vi "ltm4676a_set_runtime_config.vi"(0 "LTM4676A Runtime Config":T1={"SDC config path"=path "C:/Users/Administrator/Documents/qkocian-sandbox/demos/argus-buck-demo/instrumentstudio/sdc/pmbus_ltm4676a.sdconfig", "Output setpoint (V)"=3.3, "Voltage margin (%)"=5.0, "Voltage warn limit (%)"=7.5, "Voltage fault limit (%)"=10.0, "Switching frequency (kHz)"=650} {"Switching frequency (kHz)" items=["250"=62440, "350"=64188, "425"=64338, "500"=64488, "575"=575, "650"=650, "750"=750, "1000"=1000]; "Voltage fault limit (%)" min=0.0 max=100.0 step=1.0 format="%.1g"; "Voltage warn limit (%)" min=0.0 max=100.0 step=1.0 format="%.1g"; "Voltage margin (%)" min=0.0 max=100.0 step=1.0 format="%.1g"; "Output setpoint (V)" min=0.5 max=5.5 step=0.1}, 1 "error in (no error)":errorcluster) -> (2 "Device Control session out":refnum<class "Semiconductor Device Control.lvclass">, 3 "success?":bool, 4 "error out":errorcluster)   [LabVIEW 2021]
uses:
  <instrlib>/Semi Device Control/Semiconductor Device Control.lvclass
  controls/ltm4676a_config.ctl
  controls/ltm4676a_reg_u8.ctl
  controls/ltm4676a_reg_uids.ctl
  controls/ltm4676a_reg_u16.ctl
  <instrlib>/Semi Device Control/API/Instantiate - using IS config path.vi
  <instrlib>/Semi Device Control/API/Start.vi
  <instrlib>/Semi Device Control/API/Stop.vi
  <instrlib>/Semi Device Control/API/Destroy.vi
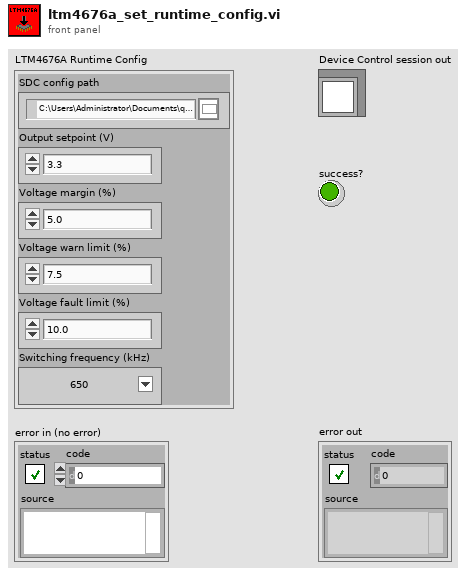
[diagram p1: front panel]
types:
  T1 = typedef "ltm4676a_config.ctl" = cluster{"SDC config path":path, "Output setpoint (V)":dbl, "Voltage margin (%)":dbl, "Voltage warn limit (%)":dbl, "Voltage fault limit (%)":dbl, "Switching frequency (kHz)":u16}
  T2 = typedef "ltm4676a_reg_uids.ctl" = string
  T3 = typedef "ltm4676a_reg_u8.ctl" = cluster{"uid":T2, "val":u8}
  T4 = typedef "ltm4676a_reg_u16.ctl" = cluster{"uid":T2, "val":u16}
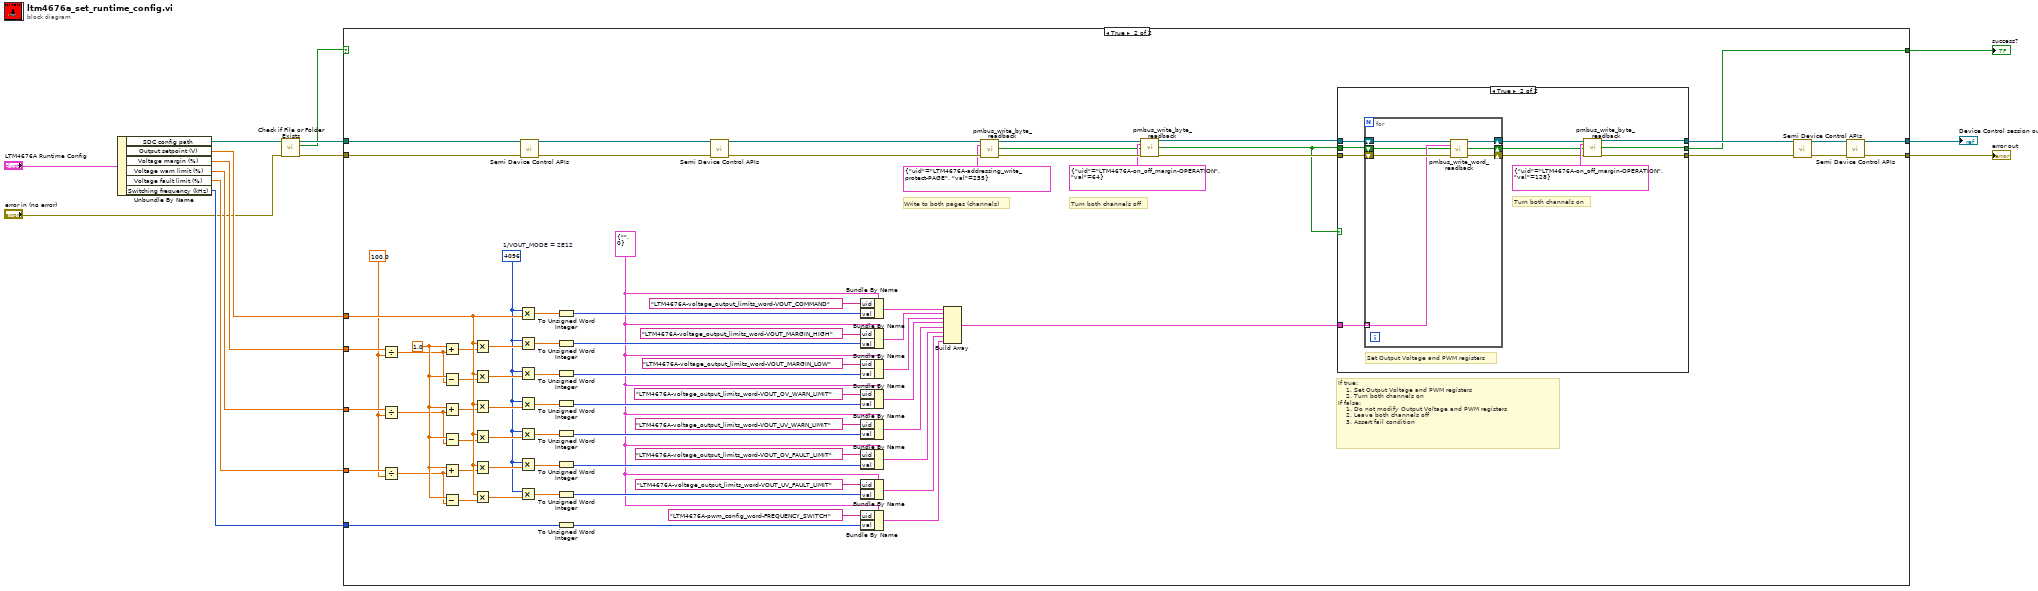
[diagram p0: block diagram]
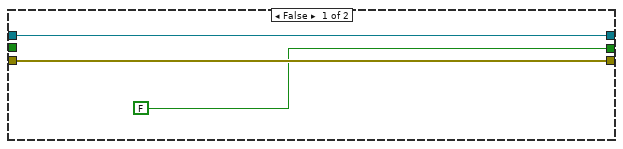
[diagram p3: hidden frame]
diagram:
  n1 = Unbundle By Name("LTM4676A Runtime Config") -> ("SDC config path"=w8:path, "Output setpoint (V)"=w9:dbl, "Voltage margin (%)"=w14:dbl, "Voltage warn limit (%)"=w13:dbl, "Voltage fault limit (%)"=w12:dbl, "Switching frequency (kHz)"=w10:u16)
  n2 = call <vilib>:"Check if File or Folder Exists.vi"("error in (no error)"="error in (no error)", "path"=w8) -> ("error out"=w6:errorcluster, "file or folder exists?"=w1:bool, "dup path"=w7:path)  [unwired: 7 in]
  n3 = case shown="True" w1 {
    selector: w1 -> [w16 _]
    tunnel: w14 -> [_ w93]
    tunnel: w13 -> [_ w92]
    tunnel: w12 -> [_ w91]
    tunnel: w10 -> [_ w90]
    tunnel: w9 -> [_ w89]
    tunnel: w7 -> [_ w88]
    tunnel: w6 -> [w15 w87]
    tunnel: [_ w86] -> w5
    tunnel: [w15 w83] -> w4
    tunnel: [w16 w77] -> w3
    frame False {
    }
    frame True {
      w17 = T4 {"uid"="", "val"=0} ("reg_u16")
      w42 = 4096  # 1/VOUT_MODE = 2E12
      w62 = 100.0 ("y")
      w66 = 1.0 ("x")
      # "If true:\n    1. Set Output Voltage and PWM registers\n    2. Turn both channels on\nIf false:\n    1. Do not modify Output Voltage and PWM registers\n    2. Leave both channels off\n    3. Assert fail condition"
      # "Turn both channels off"
      # "Write to both pages (channels)"
      n4 = Divide(x=w93, y=w62) -> (x/y=w65:dbl)
      n5 = Divide(x=w92, y=w62) -> (x/y=w64:dbl)
      n6 = Divide(x=w91, y=w62) -> (x/y=w63:dbl)
      n7 = Add(x=w66, y=w65) -> (x+y=w61:dbl)
      n8 = Subtract(x=w66, y=w65) -> (x-y=w60:dbl)
      n9 = Add(x=w66, y=w64) -> (x+y=w59:dbl)
      n10 = Subtract(x=w66, y=w64) -> (x-y=w58:dbl)
      n11 = Add(x=w66, y=w63) -> (x+y=w57:dbl)
      n12 = Subtract(x=w66, y=w63) -> (x-y=w56:dbl)
      n13 = Multiply(x=w89, y=w61) -> (x*y=w50:dbl)
      n14 = Multiply(x=w89, y=w60) -> (x*y=w51:dbl)
      n15 = Multiply(x=w89, y=w59) -> (x*y=w52:dbl)
      n16 = Multiply(x=w89, y=w58) -> (x*y=w53:dbl)
      n17 = Multiply(x=w89, y=w57) -> (x*y=w54:dbl)
      n18 = Multiply(x=w89, y=w56) -> (x*y=w55:dbl)
      n19 = Multiply(x=w42, y=w89) -> (x*y=w43:dbl)
      n20 = Multiply(x=w42, y=w50) -> (x*y=w49:dbl)
      n21 = Multiply(x=w42, y=w51) -> (x*y=w48:dbl)
      n22 = Multiply(x=w42, y=w52) -> (x*y=w47:dbl)
      n23 = Multiply(x=w42, y=w53) -> (x*y=w46:dbl)
      n24 = Multiply(x=w42, y=w54) -> (x*y=w45:dbl)
      n25 = Multiply(x=w42, y=w55) -> (x*y=w44:dbl)
      n26 = call-poly <instrlib>:"Semi Device Control APIs.vi"("IS Semi Device Control config path"=w88, "error in (no error)"=w87) -> ("Device Control session out"=w68:refnum<class "Semiconductor Device Control.lvclass">, "error out"=w67:errorcluster)  [unwired: 12 in]
      n27 = To Unsigned Word Integer(number=w43) -> (unsigned 16bit integer=w33:u16)
      n28 = To Unsigned Word Integer(number=w49) -> (unsigned 16bit integer=w32:u16)
      n29 = To Unsigned Word Integer(number=w48) -> (unsigned 16bit integer=w31:u16)
      n30 = To Unsigned Word Integer(number=w47) -> (unsigned 16bit integer=w30:u16)
      n31 = To Unsigned Word Integer(number=w46) -> (unsigned 16bit integer=w29:u16)
      n32 = To Unsigned Word Integer(number=w45) -> (unsigned 16bit integer=w28:u16)
      n33 = To Unsigned Word Integer(number=w44) -> (unsigned 16bit integer=w27:u16)
      n34 = To Unsigned Word Integer(number=w90) -> (unsigned 16bit integer=w26:u16)
      n35 = call-poly <instrlib>:"Semi Device Control APIs.vi"("Device Control session in"=w68, "error in (no error)"=w67) -> ("Device Control session out"=w79:refnum<class "Semiconductor Device Control.lvclass">, "error out"=w78:errorcluster)  [unwired: 12 in]
      n36 = Bundle By Name(cluster=w17, "uid"=T2 "LTM4676A-voltage_output_limits_word-VOUT_COMMAND" ("Register UID"), "val"=w33) -> (w25:T4)
      n37 = Bundle By Name(cluster=w17, "uid"=T2 "LTM4676A-voltage_output_limits_word-VOUT_MARGIN_HIGH" ("Register UID"), "val"=w32) -> (w24:T4)
      n38 = Bundle By Name(cluster=w17, "uid"=T2 "LTM4676A-voltage_output_limits_word-VOUT_MARGIN_LOW" ("Register UID"), "val"=w31) -> (w23:T4)
      n39 = Bundle By Name(cluster=w17, "uid"=T2 "LTM4676A-voltage_output_limits_word-VOUT_OV_WARN_LIMIT" ("Register UID"), "val"=w30) -> (w22:T4)
      n40 = Bundle By Name(cluster=w17, "uid"=T2 "LTM4676A-voltage_output_limits_word-VOUT_UV_WARN_LIMIT" ("Register UID"), "val"=w29) -> (w21:T4)
      n41 = Bundle By Name(cluster=w17, "uid"=T2 "LTM4676A-voltage_output_limits_word-VOUT_OV_FAULT_LIMIT" ("Register UID"), "val"=w28) -> (w20:T4)
      n42 = Bundle By Name(cluster=w17, "uid"=T2 "LTM4676A-voltage_output_limits_word-VOUT_UV_FAULT_LIMIT" ("Register UID"), "val"=w27) -> (w19:T4)
      n43 = Bundle By Name(cluster=w17, "uid"=T2 "LTM4676A-pwm_config_word-FREQUENCY_SWITCH" ("Register UID"), "val"=w26) -> (w18:T4)
      n44 = Build Array(w25, w24, w23, w22, w21, w20, w19, w18) -> (w80:T4[])
      n45 = call "pmbus_write_byte_readback.vi"("Device Control session in"=w79, "reg_u8"=T3 {"uid"="LTM4676A-addressing_write_protect-PAGE", "val"=255}, "error in (no error)"=w78) -> ("Device Control session out"=w76:refnum<class "Semiconductor Device Control.lvclass">, "success?"=w72:bool, "error out"=w75:errorcluster)  [unwired: 10 in]
      n46 = call "pmbus_write_byte_readback.vi"("Device Control session in"=w76, "reg_u8"=T3 {"uid"="LTM4676A-on_off_margin-OPERATION", "val"=64}, "prev success?"=w72, "error in (no error)"=w75) -> ("Device Control session out"=w71:refnum<class "Semiconductor Device Control.lvclass">, "success?"=w69:bool, "error out"=w70:errorcluster)  [unwired: 9 in]
      n47 = case shown="True" w69 {
        tunnel: [w96 w100] -> w82
        tunnel: [w95 w98] -> w81
        tunnel: w80 -> [_ w107]
        tunnel: w71 -> [w96 w106]
        tunnel: w70 -> [w95 w105]
        tunnel: [FALSE w99] -> w77
        tunnel: w69 -> [_ w97]
        frame False {
        }
        frame True {
          # "Set Output Voltage and PWM registers"
          # "Turn both channels on"
          n48 = for {
            shift-right: [w111] -> w103
            shift-left: w106 -> [w114]
            shift-right: [w110] -> w101
            shift-left: w105 -> [w113]
            tunnel: w107 -> [w109] mode=indexing
            shift-right: [w112] -> w102
            shift-left: w97 -> [w108]
            n49 = call "pmbus_write_word_readback.vi"("Device Control session in"=w114, "reg_u16"=w109, "prev success?"=w108, "error in (no error)"=w113) -> ("Device Control session out"=w111:refnum<class "Semiconductor Device Control.lvclass">, "success?"=w112:bool, "error out"=w110:errorcluster)  [unwired: 9 in]
          }
          n50 = call "pmbus_write_byte_readback.vi"("Device Control session in"=w103, "reg_u8"=T3 {"uid"="LTM4676A-on_off_margin-OPERATION", "val"=128}, "prev success?"=w102, "error in (no error)"=w101) -> ("Device Control session out"=w100:refnum<class "Semiconductor Device Control.lvclass">, "success?"=w99:bool, "error out"=w98:errorcluster)  [unwired: 9 in]
        }
      }
      n51 = call-poly <instrlib>:"Semi Device Control APIs.vi"("Device Control session in"=w82, "error in (no error)"=w81) -> ("Device Control session out"=w84:refnum<class "Semiconductor Device Control.lvclass">, "error out"=w85:errorcluster)  [unwired: 12 in]
      n52 = call-poly <instrlib>:"Semi Device Control APIs.vi"("Device Control session in"=w84, "error in (no error)"=w85) -> ("Device Control session out"=w86:refnum<class "Semiconductor Device Control.lvclass">, "error out"=w83:errorcluster)  [unwired: 12 in]
    }
  }
  "Device Control session out" <- w5
  "error out" <- w4
  "success?" <- w3
